vi "Dashboard Main.vi"() -> ()   [LabVIEW 2011]
uses:
  <vilib>/Rock Robotics/WPI/Camera/WPI_CameraImageSize.ctl
  <vilib>/Rock Robotics/WPI/DriverStation/WPI_DriverStationDigitalData.ctl
  <vilib>/Rock Robotics/WPI/Camera/WPI_CameraWhite Balance Values.ctl
  <vilib>/vision/NI_Vision_Development_Module.lvlib
panel:
  out "Taget Locked":bool
  out "RPM Error":dbl(knob) scale=-300.0..300.0
  out "Xerror To Robot":dbl(knob)=0.040581501665958725 scale=-0.1..0.1
  in  "Xerror":dbl=0.1
  out "Xcordinate":dbl=0.1 format="%_6g"
  in  "Camera Settings 3":T2={"FPS"=30, "Compression"=30, "Image Size"=enum."320x240"}
  out "Second camera":T3(plugin-control)
  out "Actual\n RPM":dbl
  out "Calculated\n RPM":dbl
  out "Best Y Value":dbl=999.0
  out "Selected\n Distance":dbl
  in  "Image \nProcessed\n Distance":dbl
  in  "Camera Settings 2":T2={"FPS"=30, "Compression"=30, "Image Size"=enum."320x240"}
  out "Turret cam Processed Image":T3(plugin-control)
  out "Turret cam Original Image":T3(plugin-control)
  in  "Annotate 2":bool=TRUE
  in  "Processing":enum32{"Intensity", "Intensity Open", "Color"}(tab)
  in  "Range":cluster{"Lower value":sgl, "Upper value":sgl}={"Lower value"=149.67392, "Upper value"=255.0} {"Lower value" scale=0.0..255.0; "Upper value" scale=0.0..255.0}
  in  "Range 2":cluster{"Lower value":sgl, "Upper value":sgl}={"Lower value"=150.0, "Upper value"=255.0} {"Lower value" scale=0.0..255.0; "Upper value" scale=0.0..255.0}
  in  "Luminance":i32=255
  in  "Saturation":i32=255
  in  "Hue":i32(knob)=65 scale=0.0..255.0
  in  "Margins":cluster{"Hue":i32, "Sat":i32, "Lum":i32}={"Hue"=9, "Sat"=40, "Lum"=19} {"Sat" scale=0.0..40.0; "Lum" scale=0.0..40.0; "Hue" scale=0.0..40.0}
  out "Target Info":T4(array[cluster])
  in  "Particle Count Limit":i32=10
  in  "Area Size Limit":i32=444
  in  "Score Limits":T5={"Rect Coverage"=76.0, "Aspect Ratio"=70.0, "X Edge Strength"=40.0, "Y Edge Strength"=60.0}
  in  "Camera Type":enum16{"206", "1011"}(ring)
  out "8 -- Battery":sgl(graph)
  out "Analog Input":sgl[](array[slide]) scale=0.0..5.0
  out "Dashboard Datatype Warning":string="Warning: The Dashboard Datatype used by the robot project and this dashboard do not match.\nSee diagram for more details."
  out "Robot IP Address":string
  out "Solenoid Output":bool[](array[boolean])
  out "PWM":cluster{u8, u8}[](array[slide])=[{0, 157}, {0, 157}, {0, 157}, {0, 157}, {0, 157}, {0, 157}, {0, 157}, {0, 157}, {0, 157}, {0, 169}] scale=1.0..255.0
  out "GPIO Output Enable":bool[](array[boolean])
  out "GPIO State":bool[](array[boolean])
  out "Relay":cluster{"Forward":bool[], "Reverse":bool[]}
  # "Analog #1"
  # "1"
  # "7"
  # "Communications"
  # "Solenoid #1"
  # "1"
  # "8"
  # "Digital #1"
  # "1"
  # "10"
  # "1"
  # "14"
  # "1"
  # "8"
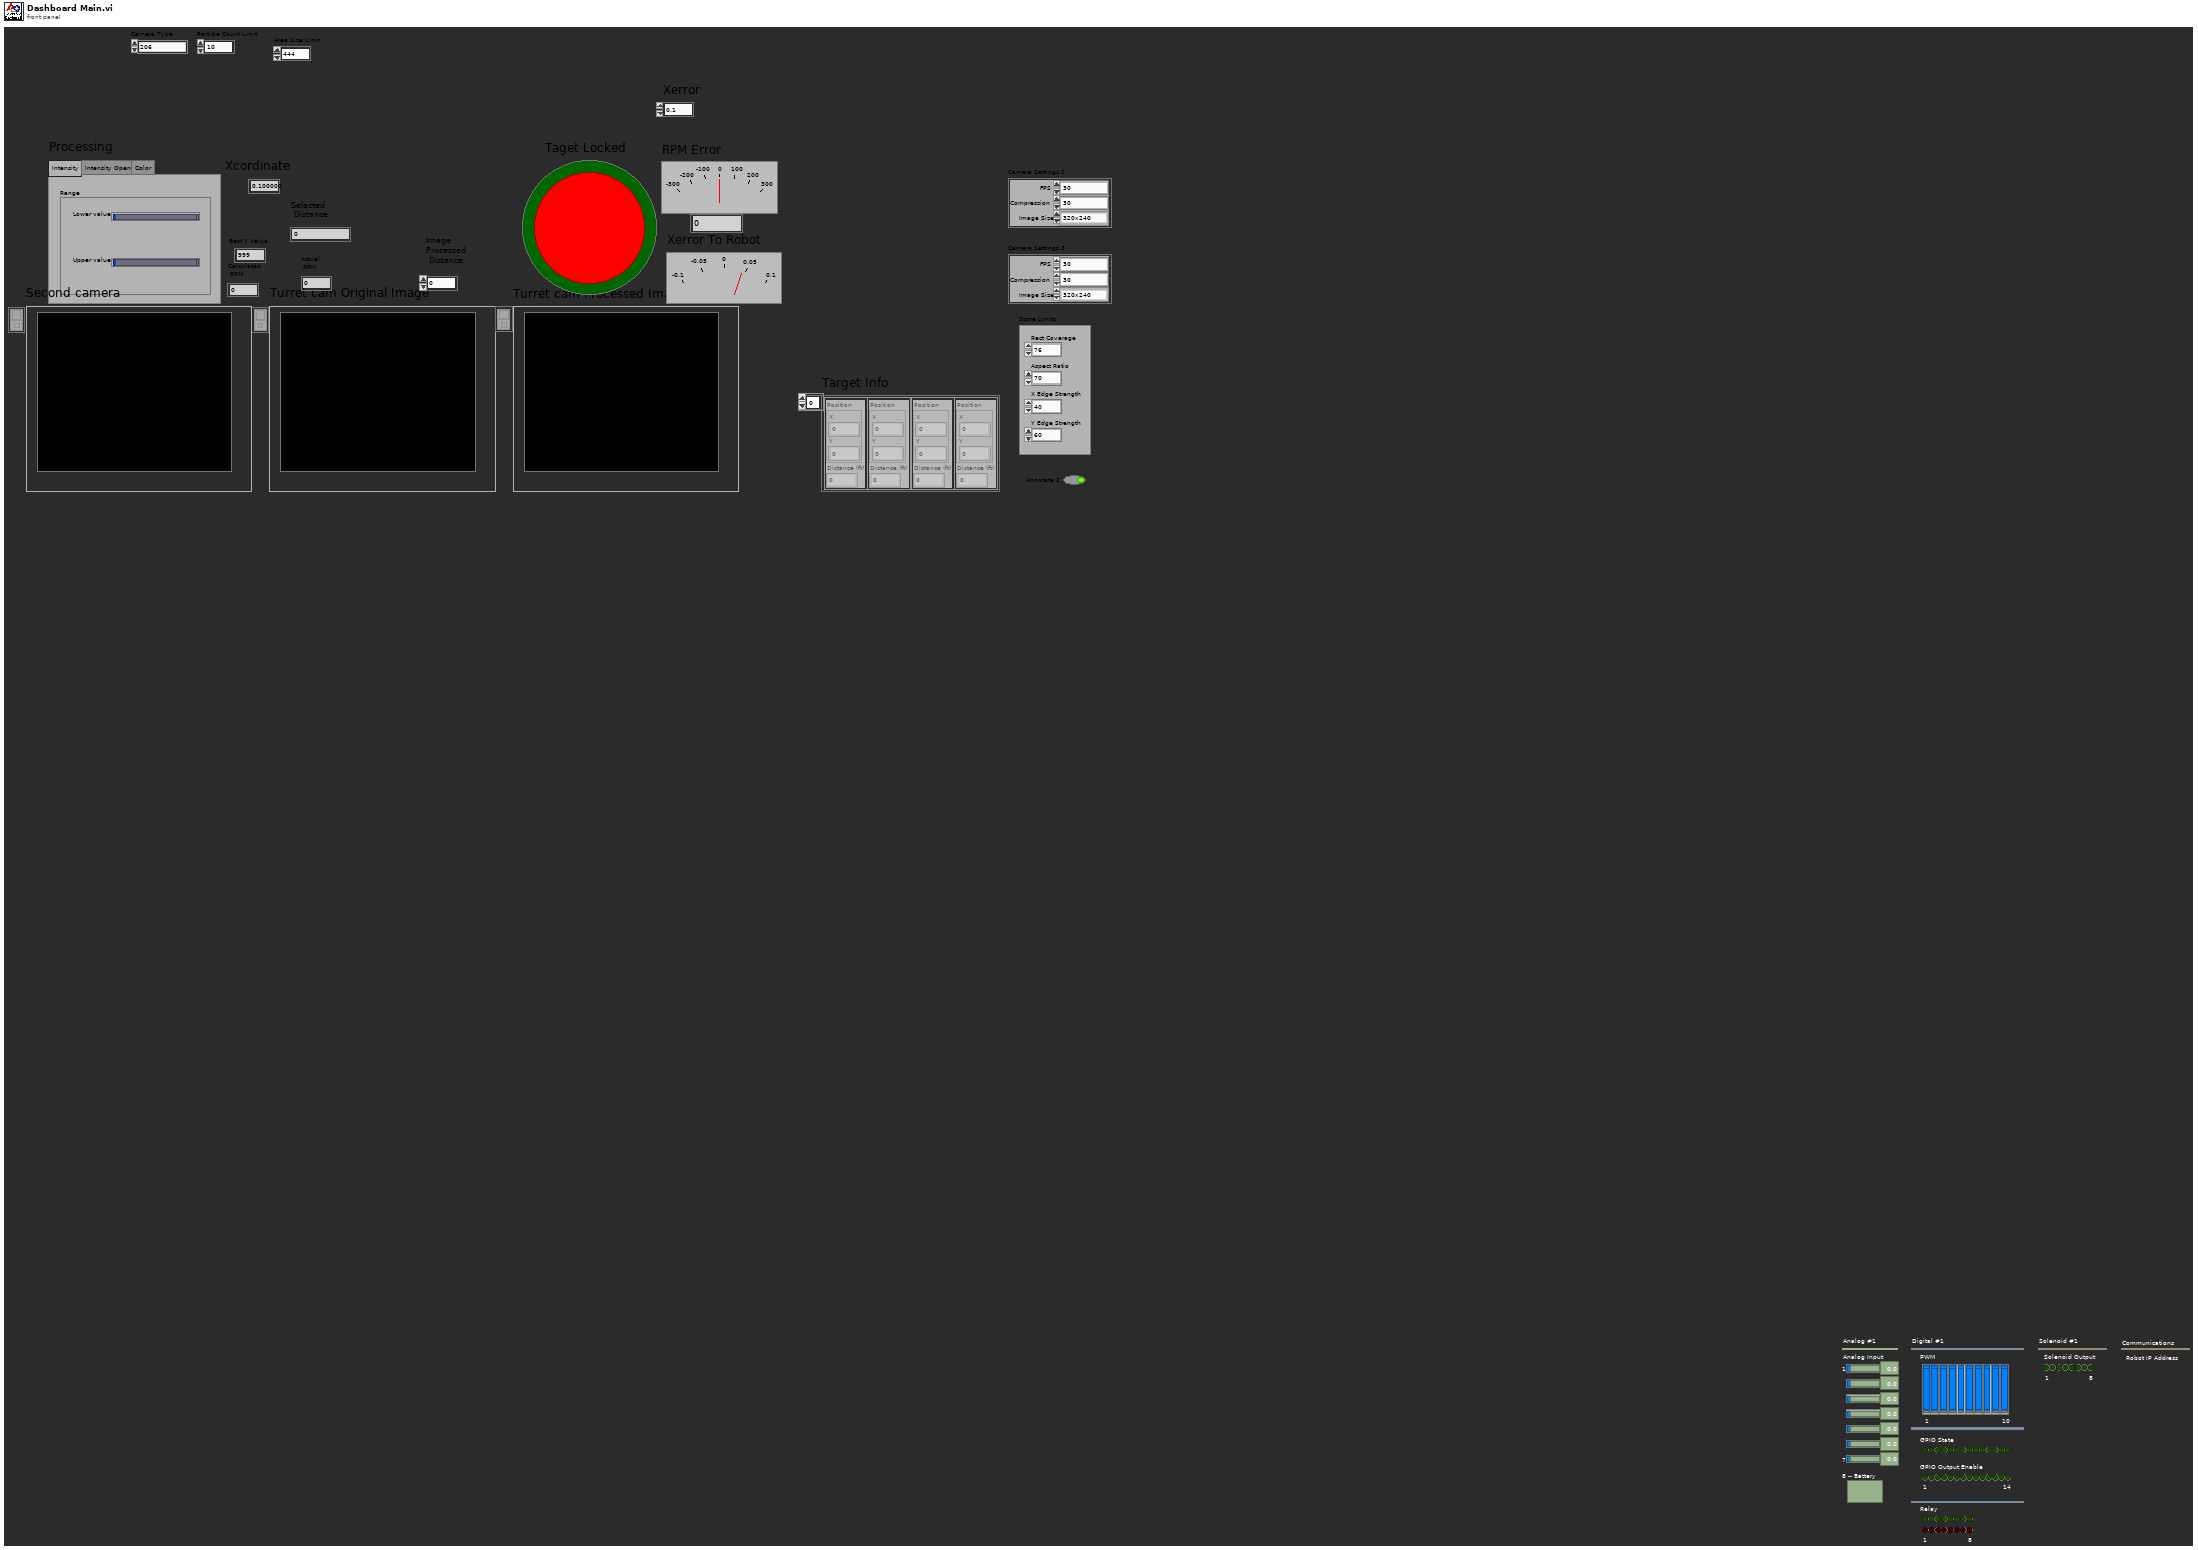
[diagram p1: front panel]
types:
  T1 = typedef "WPI_CameraImageSize.ctl" = enum16{"640x480", "320x240", "160x120"}
  T2 = cluster{"FPS":i32, "Compression":i32, "Image Size":T1}
  T3 = typedef "IMAQ Image.ctl" = refnum<image>
  T4 = cluster{"Position":cluster{"X":dbl, "Y":dbl}, "Distance (ft)":dbl}[]
  T5 = cluster{"Rect Coverage":dbl, "Aspect Ratio":dbl, "X Edge Strength":dbl, "Y Edge Strength":dbl}
  T6 = typedef "Image Type" = u32
  T7 = typedef "WPI_CameraWhite Balance Values.ctl" = enum16{"Auto", "Fixed indoor", "Fixed outdoor 1", "Fixed outdoor 2", "Fixed fluorescent 1", "Fixed fluorescent 2", "Hold current"}
  T8 = typedef "WPI_DriverStationDigitalData.ctl" = cluster{"Relay Fwd":u8, "Relay Rev":u8, "GPIO":u16, "GPIO_OE":u16, "PWM":cluster{"PWM[0]":u8, "PWM[1]":u8, "PWM[2]":u8, "PWM[3]":u8, "PWM[4]":u8, "PWM[5]":u8, "PWM[6]":u8, "PWM[7]":u8, "PWM[8]":u8, "PWM[9]":u8}}
  T9 = cluster{cluster{"AnalogModule[0]":cluster{"Channel[0]":sgl, "Channel[1]":sgl, "Channel[2]":sgl, "Channel[3]":sgl, "Channel[4]":sgl, "Channel[5]":sgl, "Channel[6]":sgl, "Channel[7]":sgl}, "AnalogModule[1]":cluster{"Channel[0]":sgl, "Channel[1]":sgl, "Channel[2]":sgl, "Channel[3]":sgl, "Channel[4]":sgl, "Channel[5]":sgl, "Channel[6]":sgl, "Channel[7]":sgl}}, cluster{"DigitalModule[0]":T8, "DigitalModule[1]":T8}, "Solenoid":u8}
  T10 = typedef "WPI_CameraDevRef.ctl" = cluster{"Camera Address":string, "CameraStatus":errorcluster, "Acquire Image Notifier":refnum<notifier>}
  T11 = cluster{"Image \nProcessed\n Distance":dbl, "Xerror ":dbl}
  T12 = enum32{"AutoM", "Close", "Dilate", "Erode", "Gradient", "Gradient out", "Gradient in", "Hit miss", "Open", "PClose", "POpen", "Thick", "Thin"}
  T13 = cluster{cluster{"Left":dbl, "Top":dbl, "Right":dbl, "Bottom":dbl}, dbl[]}[]
  T14 = cluster{"Left":dbl, "Top":dbl, "Right":dbl, "Bottom":dbl}
  T15 = cluster{"Target Center (-1 to 1)":cluster{"X":dbl, "Y":dbl}, "Distance (ft)":dbl}
  T16 = cluster{"Target Center (-1 to 1)":cluster{"X":dbl, "Y":dbl}, "Distance (ft)":dbl}[]
  T17 = cluster{"Competition mode":bool, "Robot Link":bool, "Autonomous":bool, "Enabled":bool, "E-Stop":bool}
  T18 = cluster{"AnalogModule[0]":cluster{"Channel[0]":sgl, "Channel[1]":sgl, "Channel[2]":sgl, "Channel[3]":sgl, "Channel[4]":sgl, "Channel[5]":sgl, "Channel[6]":sgl, "Channel[7]":sgl}, "AnalogModule[1]":cluster{"Channel[0]":sgl, "Channel[1]":sgl, "Channel[2]":sgl, "Channel[3]":sgl, "Channel[4]":sgl, "Channel[5]":sgl, "Channel[6]":sgl, "Channel[7]":sgl}}
  T19 = cluster{"DigitalModule[0]":T8, "DigitalModule[1]":T8}
  T20 = cluster{"Channel[0]":sgl, "Channel[1]":sgl, "Channel[2]":sgl, "Channel[3]":sgl, "Channel[4]":sgl, "Channel[5]":sgl, "Channel[6]":sgl, "Channel[7]":sgl}[]
  T21 = cluster{"Channel[0]":sgl, "Channel[1]":sgl, "Channel[2]":sgl, "Channel[3]":sgl, "Channel[4]":sgl, "Channel[5]":sgl, "Channel[6]":sgl, "Channel[7]":sgl}
  T22 = typedef "LVRectTypeDef.ctl" = cluster{"left":i16, "top":i16, "right":i16, "bottom":i16}
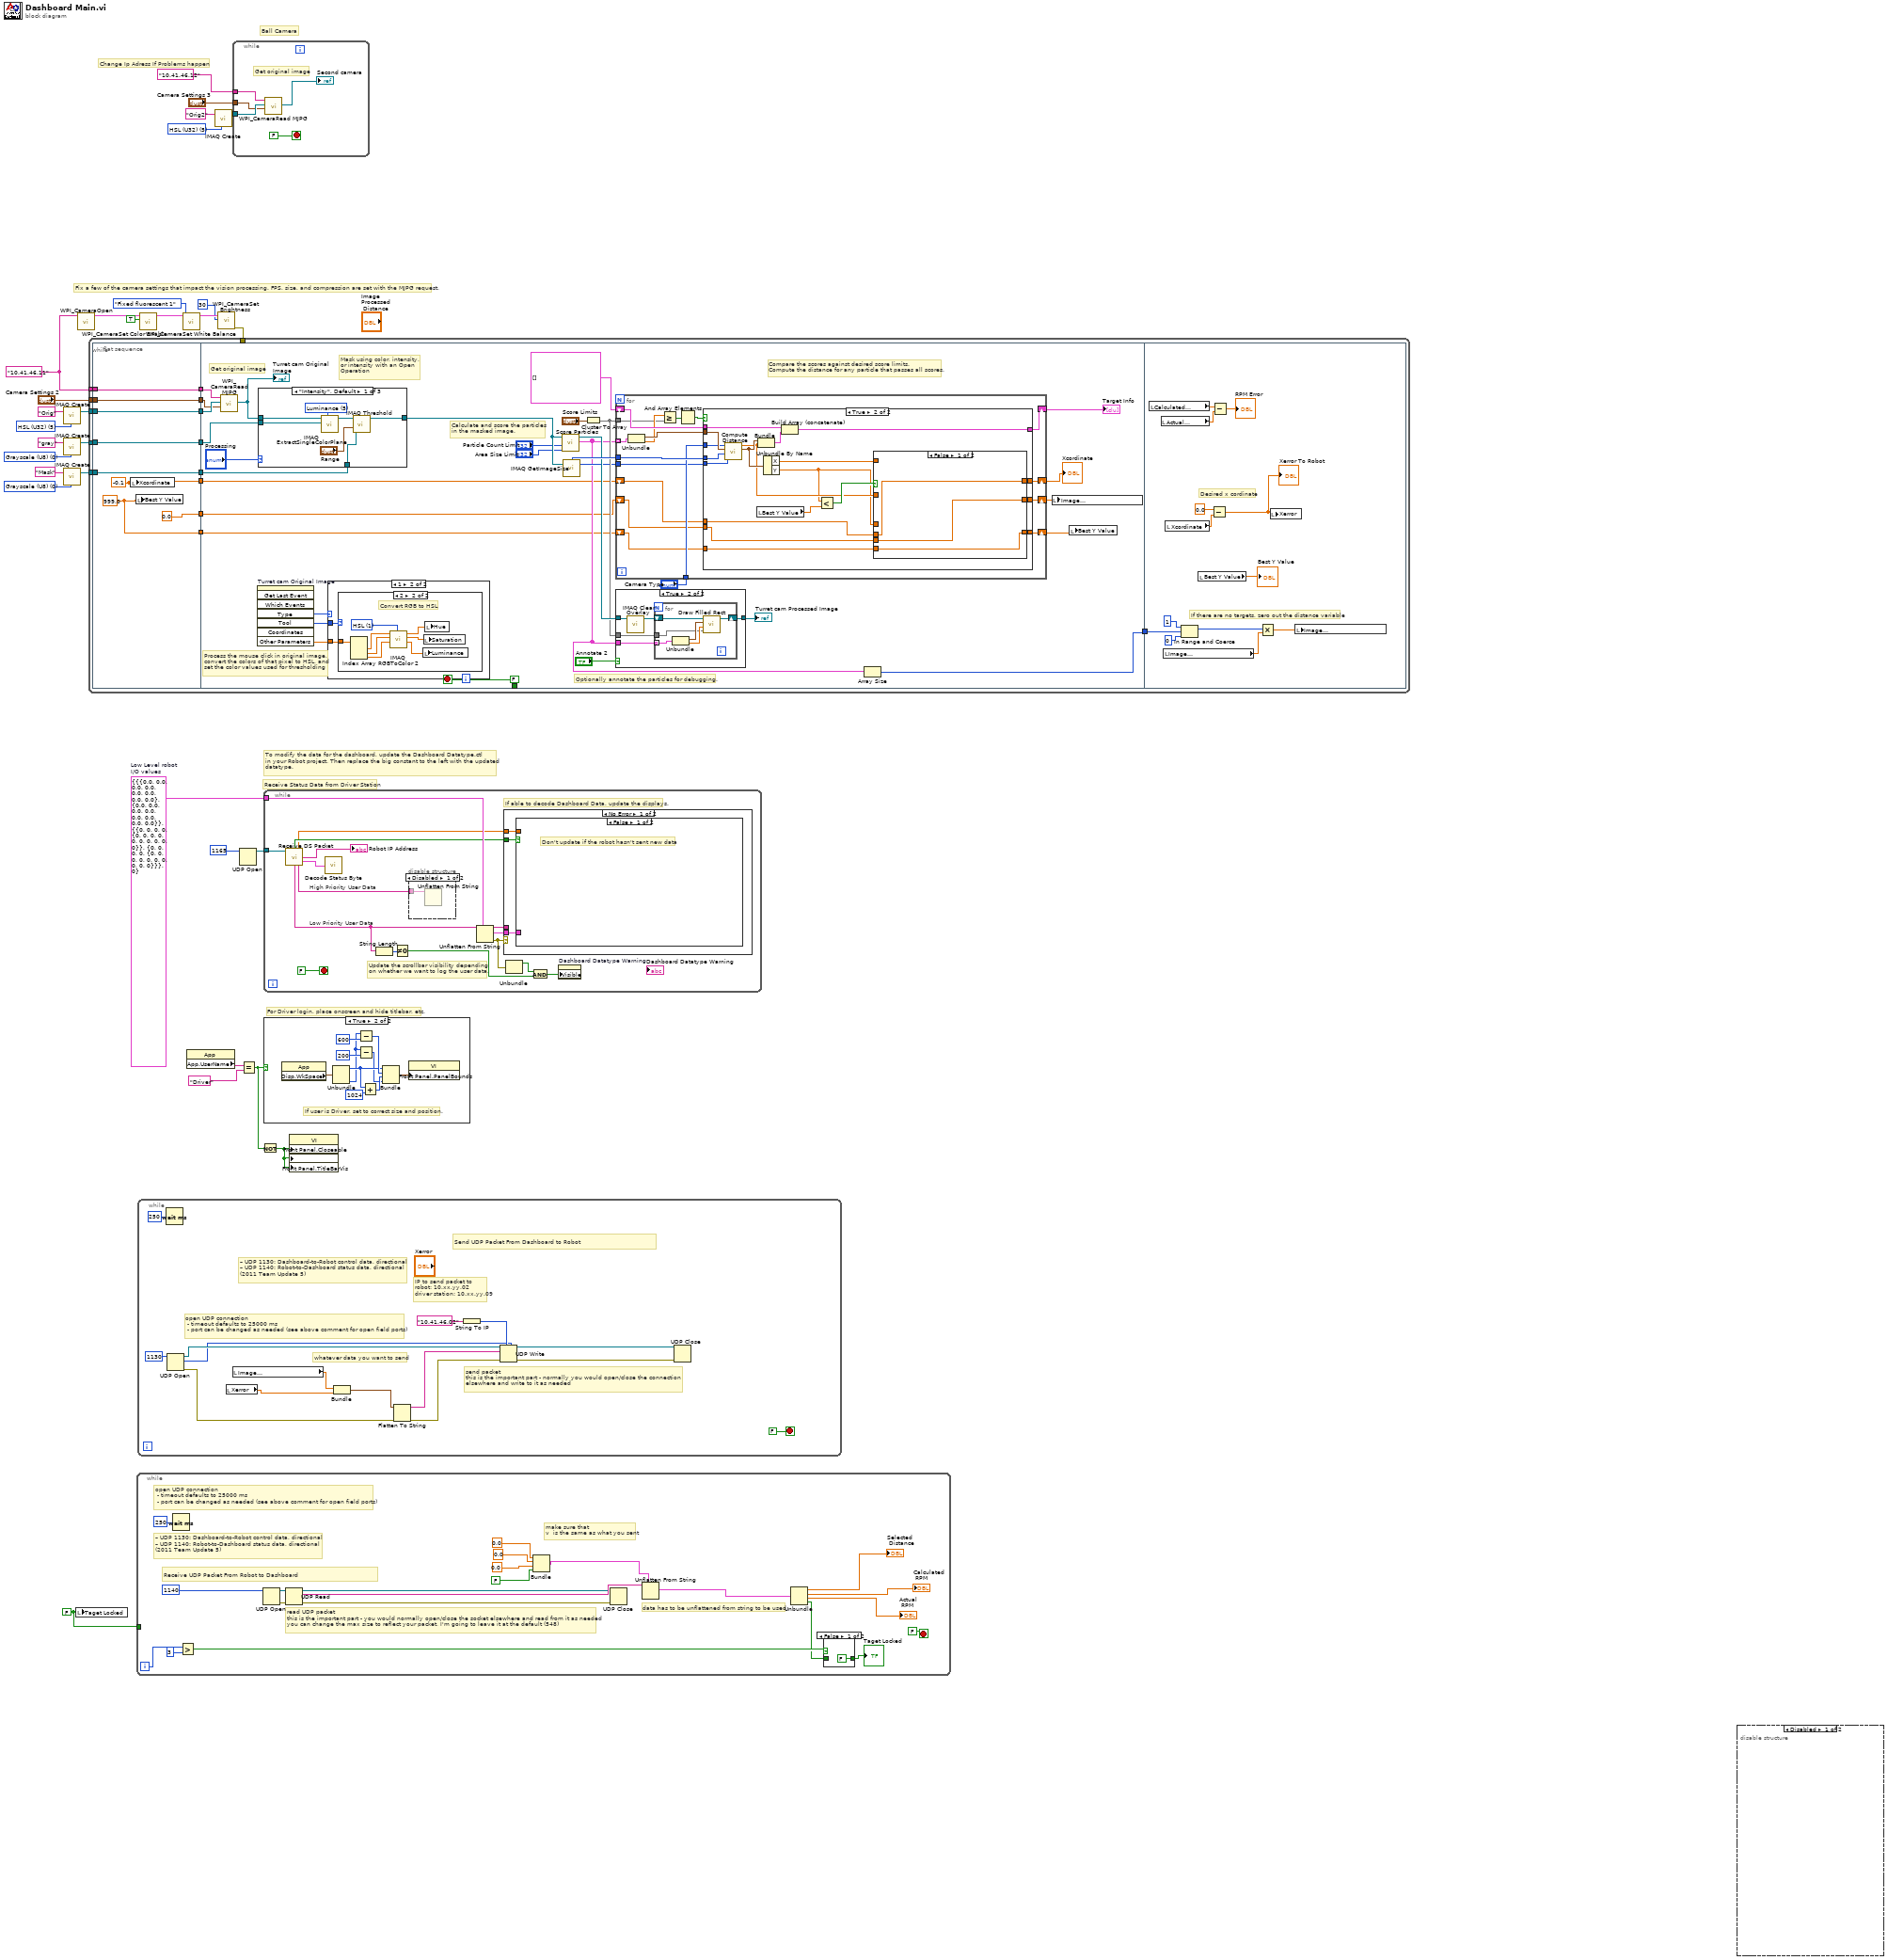
[diagram p0: block diagram]
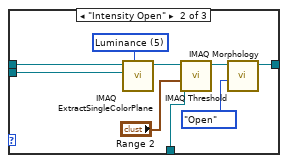
[diagram p4: hidden frame]
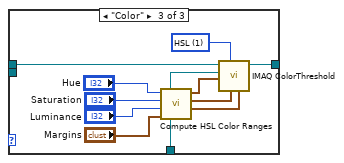
[diagram p5: hidden frame]
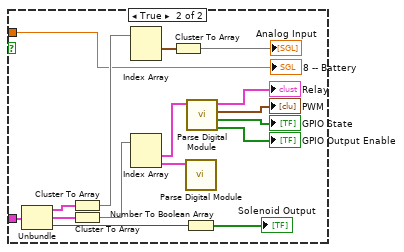
[diagram p13: hidden frame]
diagram:
  w1 = FALSE ("Taget Locked")
  w5 = T6 5 items=["Grayscale (U8)", "Grayscale (I16)", "Grayscale (SGL)", "Complex (CSG)", "RGB (U32)", "HSL (U32)", "RGB (U64)", "Grayscale (U16)"] ("Image Type")
  w7 = "10.41.46.11"
  w17 = T6 0 items=["Grayscale (U8)", "Grayscale (I16)", "Grayscale (SGL)", "Complex (CSG)", "RGB (U32)", "HSL (U32)", "RGB (U64)", "Grayscale (U16)"] ("Image Type")
  w21 = T6 5 items=["Grayscale (U8)", "Grayscale (I16)", "Grayscale (SGL)", "Complex (CSG)", "RGB (U32)", "HSL (U32)", "RGB (U64)", "Grayscale (U16)"] ("Image Type")
  w24 = T6 0 items=["Grayscale (U8)", "Grayscale (I16)", "Grayscale (SGL)", "Complex (CSG)", "RGB (U32)", "HSL (U32)", "RGB (U64)", "Grayscale (U16)"] ("Image Type")
  w25 = T9 {{"AnalogModule[0]"={"Channel[0]"=0.0, "Channel[1]"=0.0, "Channel[2]"=0.0, "Channel[3]"=0.0, "Channel[4]"=0.0, "Channel[5]"=0.0, "Channel[6]"=0.0, "Channel[7]"=0.0}, "AnalogModule[1]"={"Channel[0]"=0.0, "Channel[1]"=0.0, "Channel[2]"=0.0, "Channel[3]"=0.0, "Channel[4]"=0.0, "Channel[5]"=0.0, "Channel[6]"=0.0, "Channel[7]"=0.0}}, {"DigitalModule[0]"={"Relay Fwd"=0, "Relay Rev"=0, "GPIO"=0, "GPIO_OE"=0, "PWM"={"PWM[0]"=0, "PWM[1]"=0, "PWM[2]"=0, "PWM[3]"=0, "PWM[4]"=0, "PWM[5]"=0, "PWM[6]"=0, "PWM[7]"=0, "PWM[8]"=0, "PWM[9]"=0}}, "DigitalModule[1]"={"Relay Fwd"=0, "Relay Rev"=0, "GPIO"=0, "GPIO_OE"=0, "PWM"={"PWM[0]"=0, "PWM[1]"=0, "PWM[2]"=0, "PWM[3]"=0, "PWM[4]"=0, "PWM[5]"=0, "PWM[6]"=0, "PWM[7]"=0, "PWM[8]"=0, "PWM[9]"=0}}}, "Solenoid"=0}  # Low Level robot I/O values
  # "Change Ip Adress If Problems happen"
  # "Ball Camera"
  # "Fix a few of the camera settings that impact the vision processing. FPS, size, and compression are set with the MJPG request."
  # "For Driver login, place onscreen and hide titlebar, etc."
  # "To modify the data for the dashboard, update the Dashboard Datatype.ctl\nin your Robot project. Then replace the big constant to the left with the updated\ndatatype."
  # "Receive Status Data from Driver Station"
  n1 = call "IMAQ Create"("Image Name"="Orig", "Image Type"=w21) -> ("New Image"=w20:T3)  [unwired: 2 in, 2 out]
  n2 = call "IMAQ Create"("Image Name"="gray", "Image Type"=w24) -> ("New Image"=w19:T3)  [unwired: 2 in, 2 out]
  n3 = call "IMAQ Create"("Image Name"="Mask", "Image Type"=w17) -> ("New Image"=w16:T3)  [unwired: 2 in, 2 out]
  n4 = local write "Taget Locked"(w1) -> ()
  n5 = call <vilib>:"WPI_CameraOpen.vi"("Camera Address"=w7) -> ("CameraDevRef"=w15:T10)  [unwired: 9 in, 1 out]
  n6 = while {
    tunnel: w1 -> [_]
    i -> [w36]
    stop <- FALSE stop-if-true
    # "make sure that\nv  is the same as what you sent"
    # "data has to be unflattened from string to be used"
    # "read UDP packet\nthis is the important part - you would normally open/close the socket elsewhere and read from it as needed\nyou can change the max size to reflect your packet, I'm going to leave it at the default (548)"
    # "open UDP connection\n - timeout defaults to 25000 ms\n - port can be changed as needed (see above comment for open field ports)"
    # "– UDP 1130: Dashboard-to-Robot control data, directional\n– UDP 1140: Robot-to-Dashboard status data, directional\n(2011 Team Update 5)"
    # "Receive UDP Packet From Robot to Dashboard"
    n7 = Wait (ms)(milliseconds to wait=u32 250) -> ()  [unwired: 1 out]
    n8 = Greater?(x=w36, y=3) -> (0:w34:bool)
    n9 = UDP Open(11:u16 1140 ("port")) -> (port=w52:refnum<k16>, 0:w51:errorcluster)  [unwired: 1 in, 4 out]
    n10 = UDP Read(connection ID=w52, 8:w51) -> (data out=w50:string, error out=w47:errorcluster, 3:w48:refnum<k16>)  [unwired: 4 out]
    n11 = Bundle(0.0, 0.0, 0.0, FALSE) -> (w41:cluster{dbl, dbl, dbl, bool})  [unwired: 1 in]
    n12 = UDP Close(connection ID=w48, 8:w47) -> ()  [unwired: 2 out]
    n13 = Unflatten From String(type=w41, binary string=w50) -> (value=w49:cluster{dbl, dbl, dbl, bool})  [unwired: 1 in, 4 out]
    n14 = Unbundle(w49) -> (→"Selected\n Distance":dbl, →"Calculated\n RPM":dbl, →"Actual\n RPM":dbl, w33:bool)
    n15 = case shown="False" w34 {
      tunnel: [FALSE w55] -> w32
      tunnel: w33 -> [_ w55]
      frame False {
      }
      frame True {
      }
    }
    "Taget Locked" <- w32
  }
  n16 = while {
    stop <- FALSE stop-if-true
    # "send packet\nthis is the important part - normally you would open/close the connection \nelsewhere and write to it as needed"
    # "whatever data you want to send"
    # "IP to send packet to \nrobot: 10.xx.yy.02\ndriver station: 10.xx.yy.09"
    # "open UDP connection\n - timeout defaults to 25000 ms\n - port can be changed as needed (see above comment for open field ports)"
    # "Send UDP Packet From Dashboard to Robot"
    # "– UDP 1130: Dashboard-to-Robot control data, directional\n– UDP 1140: Robot-to-Dashboard status data, directional\n(2011 Team Update 5)"
    n17 = Wait (ms)(milliseconds to wait=u32 250) -> ()  [unwired: 1 out]
    n18 = UDP Open(11:u16 1130 ("port")) -> (port=w61:refnum<k16>, 0:w59:errorcluster, 2:w60:u16)  [unwired: 1 in, 3 out]
    n19 = local read "Xerror"() -> (w57:dbl)
    n20 = local read "Image \nProcessed\n Distance"() -> (w58:dbl)
    n21 = Bundle("Image \nProcessed\n Distance"=w58, "Xerror"=w57) -> (w56:T11)  [unwired: 1 in]
    n22 = Flatten To String(anything=w56, error in (no error)=w59) -> (data string=w66:string, error out=w67:errorcluster)  [unwired: 3 out]
    n23 = String To IP(1:"10.41.46.02") -> (0:w68:u32)
    n24 = UDP Write(address=w68, port or service name=w60, connection ID=w61, data in=w66, 8:w67) -> (error out=w64:errorcluster, 3:w65:refnum<k16>)  [unwired: 1 out]
    n25 = UDP Close(connection ID=w65, 8:w64) -> ()  [unwired: 2 out]
  }
  n26 = call <vilib>:"WPI_CameraSet Color Enable.vi"("Color Enabled"=TRUE, "CameraDevRef"=w15) -> ("CameraDevRef Out"=w13:T10)  [unwired: 8 in, 1 out]
  n27 = call <vilib>:"WPI_CameraSet White Balance.vi"("White Balance"=WPI_CameraWhite_Balance_Values."Fixed fluorescent 1", "CameraDevRef"=w13) -> ("CameraDevRef Out"=w11:T10)  [unwired: 8 in, 1 out]
  n28 = property class="App"() -> ("App.UserName"=w28:string)  [unwired: 2 in, 2 out]
  n29 = call "IMAQ Create"("Image Name"="Orig2", "Image Type"=w5) -> ("New Image"=w4:T3)  [unwired: 2 in, 2 out]
  n30 = call <vilib>:"WPI_CameraSet Brightness.vi"("Brightness"=30, "CameraDevRef"=w11) -> ("error out"=w9:errorcluster)  [unwired: 8 in, 1 out]
  n31 = while {
    tunnel: w20 -> [w82]
    tunnel: w19 -> [w85]
    tunnel: w16 -> [w84]
    tunnel: w7 -> [w81]
    tunnel: w9 -> [_]
    tunnel: "Camera Settings 2" -> [w80]
    stop <- w83 stop-if-true
    n32 = flat-sequence {
      tunnel: w80 -> [w89]
      tunnel: w81 -> [w90]
      tunnel: w82 -> [w91]
      tunnel: w84 -> [w92]
      tunnel: w85 -> [w93]
      tunnel: [w93] -> w79
      tunnel: [w92] -> w78
      tunnel: [w91] -> w77
      tunnel: [w90] -> w76
      tunnel: [w89] -> w75
      tunnel: [w88] -> w73
      tunnel: [w87] -> w72
      tunnel: [0.0] -> w71
      tunnel: [FALSE] -> w83
      tunnel: w79 -> [w125]
      tunnel: w78 -> [w124]
      tunnel: w77 -> [w116]
      tunnel: w76 -> [w114]
      tunnel: w75 -> [w102]
      tunnel: [w100] -> w74
      tunnel: w73 -> [w96]
      tunnel: w72 -> [w95]
      tunnel: w71 -> [w94]
      tunnel: w74 -> [w224]
      frame #0 {
        w87 = 999.0
        w88 = -0.1 ("Xcordinate")
        n33 = local write "Xcordinate"(w88) -> ()
        n34 = local write "Best Y Value"(w87) -> ()
      }
      frame #1 {
        # "Optionally annotate the particles for debugging."
        # "Compare the scores against desired score limits.\nCompute the distance for any particle that passes all scores."
        # "Process the mouse click in original image,\nconvert the colors of that pixel to HSL, and\nset the color values used for thresholding"
        # "Calculate and score the particles\nin the masked image."
        # "Mask using color, intensity,\nor intensity with an Open\nOperation"
        # "Get original image"
        n35 = call <vilib>:"WPI_CameraRead MJPG.vi"("Camera Settings"=w102, "Image"=w116, "address"=w114) -> ("Image Out"=w115:T3)  [unwired: 7 in, 1 out]
        "Turret cam Original Image" <- w115
        n36 = invoke on="Turret cam Original Image" class="ImageControl" method="Get Last Event"() -> ("Type"=w118:i32, "Tool"=w119:i32, "Other Parameters"=w120:sgl[])  [unwired: 8 in, 5 out]
        n37 = case shown="\"Intensity\", Default" "Processing" {
          tunnel: w115 -> [w144 w153 w164]
          tunnel: w125 -> [w143 w152 _]
          tunnel: w124 -> [w141 w150 w163]
          tunnel: [w139 w146 w162] -> w107
          frame "Intensity", Default {
            w138 = 5 items=["Red", "Green", "Blue", "Hue", "Saturation", "Luminance", "Value", "Intensity"] ("Color Plane")
            n38 = call "IMAQ ExtractSingleColorPlane"("Color Plane"=w138, "Image Dst"=w143, "Image Src"=w144) -> ("Image Dst Out"=w142:T3)  [unwired: 1 in, 7 out]
            n39 = call "IMAQ Threshold"("Range"="Range", "Image Dst"=w141, "Image Src"=w142) -> ("Image Dst Out"=w139:T3)  [unwired: 3 in, 5 out]
          }
          frame "Intensity Open" {
            w145 = 5 items=["Red", "Green", "Blue", "Hue", "Saturation", "Luminance", "Value", "Intensity"] ("Color Plane")
            n40 = call "IMAQ ExtractSingleColorPlane"("Color Plane"=w145, "Image Dst"=w152, "Image Src"=w153) -> ("Image Dst Out"=w151:T3)  [unwired: 1 in, 7 out]
            n41 = call "IMAQ Threshold"("Range"="Range 2", "Image Dst"=w150, "Image Src"=w151) -> ("Image Dst Out"=w147:T3)  [unwired: 3 in, 5 out]
            n42 = call "IMAQ Morphology"("Operation"=T12."Open", "Image Src"=w147) -> ("Image Dst Out"=w146:T3)  [unwired: 8 in, 1 out]
          }
          frame "Color" {
            w161 = u16 1 items=["RGB", "HSL", "HSV", "HSI"] ("Color Mode")
            n43 = call "Compute HSL Color Ranges.vi"("Margins"="Margins", "Luminance"="Luminance", "Saturation"="Saturation", "Hue"="Hue") -> ("Lum Range"=w158:cluster{i32, i32}, "Sat Range"=w159:cluster{i32, i32}, "Hue Range"=w160:cluster{i32, i32})  [unwired: 5 in]
            n44 = call "IMAQ ColorThreshold"("Blue or Luma or Val or Inten Range"=w158, "Green or Sat Range"=w159, "Color Mode"=w161, "Red or Hue Range"=w160, "Image Dst"=w163, "Image Src"=w164) -> ("Image Dst Out"=w162:T3)  [unwired: 4 in, 1 out]
          }
        }
        n45 = case shown="1" w118 {
          tunnel: w119 -> [_ w212]
          tunnel: w120 -> [_ w211]
          frame 0, Default {
          }
          frame 1 {
            n46 = case shown="2" w212 {
              tunnel: w211 -> [_ w220]
              frame Default {
              }
              frame 2 {
                w219 = u16 1 items=["RGB", "HSL", "HSV", "HSI", "CIE L*a*b*", "CIE XYZ"] ("Color Mode")
                # "Convert RGB to HSL"
                n47 = Index Array(array=w220) -> (element #1=w218:sgl, element #2=w216:sgl, element #3=w214:sgl)  [unwired: 3 in]
                n48 = call "IMAQ RGBToColor 2"("Color Mode"=w219, "Blue value"=w214, "Green value"=w216, "Red value"=w218) -> ("Blue or Luma or Val or Inten or Z or b*value"=w213:dbl, "Green or Sat or Y or a* value"=w215:dbl, "Red or Hue or X or L* value"=w217:dbl)  [unwired: 4 in, 1 out]
                n49 = local write "Luminance"(w213) -> ()
                n50 = local write "Saturation"(w215) -> ()
                n51 = local write "Hue"(w217) -> ()
              }
            }
          }
        }
        n52 = call "Score Particles.vi"("Area Size Limit"="Area Size Limit", "Particle Count Limit"="Particle Count Limit", "Image Refnum in"=w107) -> ("Scored Particle Info"=w101:T13, "Image Refnum out"=w113:T3)  [unwired: 7 in]
        n53 = call "IMAQ GetImageSize"("Image"=w107) -> ("Y Resolution"=w103:i32, "X Resolution"=w117:i32)  [unwired: 3 in, 1 out]
        n54 = Cluster To Array(cluster="Score Limits") -> (array=w108:dbl[])
        n55 = for {
          shift-right: [w180] -> w121
          shift-left: T4 [] -> [w181]
          tunnel: w117 -> [w179]
          tunnel: w101 -> [w177] mode=indexing
          tunnel: w108 -> [w172]
          tunnel: "Camera Type" -> [w176]
          tunnel: w103 -> [w171]
          shift-right: [w170] -> w99
          shift-left: w96 -> [w167]
          shift-right: [w169] -> w98
          shift-left: w94 -> [w166]
          shift-right: [w168] -> w97
          shift-left: w95 -> [w165]
          n56 = Unbundle(w177) -> (w178:T14, w173:dbl[])
          n57 = Greater Or Equal?(x=w173, y=w172) -> (x >= y?=w175:bool[])
          n58 = And Array Elements(Boolean array=w175) -> (logical AND=w174:bool)
          n59 = case shown="True" w174 {
            tunnel: w181 -> [w185 w204]
            tunnel: [w185 w203] -> w180
            tunnel: w178 -> [_ w200]
            tunnel: w179 -> [_ w201]
            tunnel: w176 -> [_ w199]
            tunnel: w171 -> [_ w198]
            tunnel: [w184 w191] -> w170
            tunnel: [w183 w190] -> w169
            tunnel: [w182 w189] -> w168
            tunnel: w167 -> [w184 w188]
            tunnel: w166 -> [w183 w187]
            tunnel: w165 -> [w182 w186]
            frame False {
            }
            frame True {
              n60 = call "Compute Distance.vi"("Y Image Resolution"=w198, "X Image Resolution"=w201, "Bounding Box"=w200, "Camera Type"=w199) -> ("Target Center (-1 to 1)"=w195:cluster{"X":dbl, "Y":dbl}, "Distance (ft)"=w194:dbl)  [unwired: 6 in]
              n61 = local read "Best Y Value"() -> (w197:dbl)
              n62 = Bundle("Target Center (-1 to 1)"=w195, "Distance (ft)"=w194) -> (w202:T15)  [unwired: 1 in]
              n63 = Unbundle By Name(w195) -> ("X"=w193:dbl, "Y"=w192:dbl)
              n64 = Build Array (concatenate)(w204, w202) -> (w203:T16)
              n65 = Less?(x=w192, y=w197) -> (x < y?=w196:bool)
              n66 = case shown="False" w196 {
                tunnel: w194 -> [_ w209]
                tunnel: w193 -> [_ w210]
                tunnel: w192 -> [_ w208]
                tunnel: [w207 w210] -> w191
                tunnel: [w206 w209] -> w190
                tunnel: [w205 w208] -> w189
                tunnel: w188 -> [w207 _]
                tunnel: w187 -> [w206 _]
                tunnel: w186 -> [w205 _]
                frame False {
                }
                frame True {
                }
              }
            }
          }
        }
        "Target Info" <- w121
        "Xcordinate" <- w99
        n67 = case shown="True" "Annotate 2" {
          tunnel: w113 -> [w126 w131]
          tunnel: [w126 w130] -> w110
          tunnel: w101 -> [_ w128]
          tunnel: w108 -> [_ w127]
          frame False {
          }
          frame True {
            n68 = call "IMAQ Clear Overlay"("Image"=w131) -> ("Image Out"=w129:T3)  [unwired: 2 in, 8 out]
            n69 = for {
              shift-right: [w136] -> w130
              shift-left: w129 -> [w137]
              tunnel: w128 -> [w133] mode=indexing
              tunnel: w127 -> [w132]
              n70 = Unbundle(w133) -> (w134:T14, w135:dbl[])
              n71 = call "Draw Filled Rect.vi"("Limits"=w132, "Scores"=w135, "Bounding Box"=w134, "image in"=w137) -> ("image out"=w136:T3)  [unwired: 7 in]
            }
          }
        }
        "Turret cam Processed Image" <- w110
        n72 = Array Size(array=w101) -> (size(s)=w100:i32)
        n73 = local write "Image \nProcessed\n Distance"(w98) -> ()
        n74 = local write "Best Y Value"(w97) -> ()
      }
      frame #2 {
        # "If there are no targets, zero out the distance variable"
        # "Desired x cordinate"
        n75 = local read "Calculated\n RPM"() -> (w231:dbl)
        n76 = local read "Actual\n RPM"() -> (w230:dbl)
        n77 = local read "Image \nProcessed\n Distance"() -> (w222:dbl)
        n78 = local read "Xcordinate"() -> (w233:dbl)
        n79 = In Range and Coerce(upper limit=1, x=w224, lower limit=0) -> (coerced(x)=w223:i32)  [unwired: 1 out]
        n80 = local read "Best Y Value"() -> (→"Best Y Value":dbl)
        n81 = Subtract(x=0.0, y=w233) -> (x-y=w228:dbl)
        "Xerror To Robot" <- w228
        n82 = Subtract(x=w231, y=w230) -> (x-y=→"RPM Error":dbl)
        n83 = Multiply(x=w223, y=w222) -> (x*y=w221:dbl)
        n84 = local write "Xerror"(w228) -> ()
        n85 = local write "Image \nProcessed\n Distance"(w221) -> ()
      }
    }
  }
  n86 = while {
    tunnel: w4 -> [w237]
    tunnel: "10.41.46.12" -> [w235]
    tunnel: "Camera Settings 3" -> [w234]
    stop <- FALSE stop-if-true
    # "Get original image"
    n87 = call <vilib>:"WPI_CameraRead MJPG.vi"("Camera Settings"=w234, "Image"=w237, "address"=w235) -> ("Image Out"=→"Second camera":T3)  [unwired: 7 in, 1 out]
  }
  n88 = UDP Open(11:u16 1165 ("port")) -> (port=w30:refnum<k16>)  [unwired: 2 in, 4 out]
  n89 = Equal?(x=w28, y="Driver") -> (x = y?=w27:bool)
  n90 = Not(x=w27) -> (.not. x?=w26:bool)
  n91 = while {
    tunnel: w30 -> [w252]
    tunnel: w25 -> [w251]
    stop <- FALSE stop-if-true
    # "High Priority User Data"
    # "Low Priority User Data"
    # "Update the scrollbar visibility depending\non whether we want to log the user data."
    # "If able to decode Dashboard Data, update the displays."
    n92 = call "Receive DS Packet.vi"("Recv Socket"=w252) -> ("New Dashboard Data"=w248:bool, "Battery"=w239:sgl, "Robot IP Address"=→"Robot IP Address":string, "Status"=w253:T17, "Low Priority User Data"=w241:string, "High Priority User Data"=w240:string)  [unwired: 1 in, 8 out]
    n93 = call "Decode Status Byte.vi"("Status Byte"=w253) -> ()  [unwired: 2 out]
    n94 = String Length(string=w241) -> (length=w243:i32)
    n95 = Not Equal To 0?(x=w243) -> (x != 0?=w246:bool)
    n96 = disable-structure shown="Disabled" {
      disable-tunnel: w240 -> [w255 _]
      frame Disabled {
        n97 = Unflatten From String(binary string=w255) -> ()  [unwired: 2 in, 5 out]
      }
      frame Enabled {
      }
    }
    n98 = Unflatten From String(type=w251, binary string=w241) -> (rest of the binary string=w244:string, value=w250:T9, error out=w249:errorcluster)  [unwired: 1 in, 2 out]
    n99 = case shown="No Error" w249 {
      tunnel: w250 -> [w258 _]
      tunnel: w248 -> [w257 _]
      tunnel: w244 -> [_ _]
      tunnel: w239 -> [w256 _]
      frame No Error {
        n100 = case shown="False" w257 {
          tunnel: w258 -> [_ w265]
          tunnel: w256 -> [_ w259]
          frame False {
            # "Don't update if the robot hasn't sent new data"
          }
          frame True {
            n101 = Unbundle(w265) -> (w262:T18, w263:T19, "Solenoid"=w264:u8)
            n102 = Cluster To Array(cluster=w262) -> (array=w273:T20)
            n103 = Cluster To Array(cluster=w263) -> (array=w272:T8[])
            n104 = Index Array(array=w273) -> (element #1=w260:T21)  [unwired: 2 in, 1 out]
            n105 = Index Array(array=w272) -> (element #1=w271:T8, element #2=w266:T8)  [unwired: 2 in]
            n106 = Cluster To Array(cluster=w260) -> (array=→"Analog Input":sgl[])
            n107 = call "Parse Digital Module.vi"("DigitalModule"=w266) -> ()  [unwired: 11 out]
            n108 = Number To Boolean Array(number=w264) -> (Boolean array=→"Solenoid Output":bool[])
            n109 = call "Parse Digital Module.vi"("DigitalModule"=w271) -> ("GPIO Output Enable"=→"GPIO Output Enable":bool[], "GPIO State"=→"GPIO State":bool[], "PWM"=→"PWM":cluster{u8, u8}[], "Relay"=→"Relay":cluster{"Forward":bool[], "Reverse":bool[]})  [unwired: 7 out]
            "8 -- Battery" <- w259
          }
        }
      }
      frame Error {
        # "Your datatypes don't match. The Dashboard Datatype.ctl in your Robot project\nand the big constant to the left of the loop need to match."
      }
    }
    n110 = Unbundle(w249) -> ("status"=w245:bool)  [unwired: 2 out]
    n111 = And(x=w245, y=w246) -> (x .and. y?=w247:bool)
    n112 = property on="Dashboard Datatype Warning" class="Str"("Visible"=w247) -> ()  [unwired: 2 in, 2 out]
  }
  n113 = case shown="True" w27 {
    frame False {
    }
    frame True {
      # "If user is Driver, set to correct size and position."
      n114 = property class="App"() -> ("Disp.WkSpace"=w284:T22)  [unwired: 2 in, 2 out]
      n115 = Unbundle(w284) -> ("left"=w279:i16, "bottom"=w275:i16)  [unwired: 2 out]
      n116 = Subtract(x=w275, y=600) -> (x-y=w281:i32)
      n117 = Subtract(x=w275, y=200) -> (x-y=w276:i32)
      n118 = Add(x=w279, y=1024) -> (x+y=w280:i32)
      n119 = Bundle("left"=w279, w281, w280, w276) -> (w283:cluster{"left":i16, i32, i32, i32})  [unwired: 1 out]
      n120 = property class="VI"("Front Panel.PanelBounds"=w283) -> ()  [unwired: 2 in, 2 out]
    }
  }
  n121 = property class="VI"("Front Panel.Closeable"=w26, "Front Panel.Minimizeable"=w26, "Front Panel.TitleBarVis"=w26) -> ()  [unwired: 2 in, 2 out]
  n122 = disable-structure shown="Disabled" {
    frame Disabled {
    }
    frame Enabled {
    }
  }
